vi "UnitatsStrings.vi"(1 "UnidadesCelula":i32[](array[numeric])) -> (0 "StringUnidades":string)   [LabVIEW 2014]
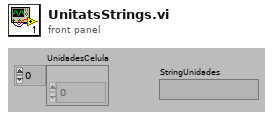
[diagram p1: front panel]
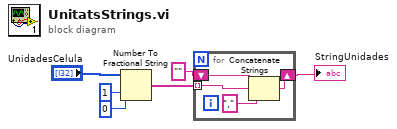
[diagram p0: block diagram]
diagram:
  n1 = Number To Fractional String(number="UnidadesCelula", width (-)=i16 1, precision (6)=i16 0) -> (F-format string=w2:string[])  [unwired: 1 in]
  n2 = for {
    tunnel: w2 -> [w10] mode=indexing
    shift-right: [w9] -> w6
    shift-left: "" -> [w7]
    n3 = Concatenate Strings(w7, w10, "," ("string")) -> (w9:string)
  }
  "StringUnidades" <- w6
